vi "rs3 start all 2.vi"(7 "capacity":i32=2, 8 "error in (no error)":errorcluster, 9 "Count of Streams":i32=2, 10 "Sensor in":u64, 11 "Stream profile array":u64[](array[numeric])) -> (0 "error out":errorcluster, 2 "sensor out":u64, 3 "Config Error":string, 5 "queue out":u64)   [LabVIEW 2019, in "libRealSense3.lvlib"]
doc: "STARTs all the streams for the selected sensor.\n\nInput:\nStream profile array The array containing the handles to the Profiles you want to stream\nCount Number of streams in the array\nCapacity Should generally exceed or equal the count."
uses:
  libRealSense3.lvlib
panel:
  out "Sensor":dbl
  out "Stream Count":dbl
  # "RS3 Start all"
  # "(C) Intel Corp 2017,  AGJ"
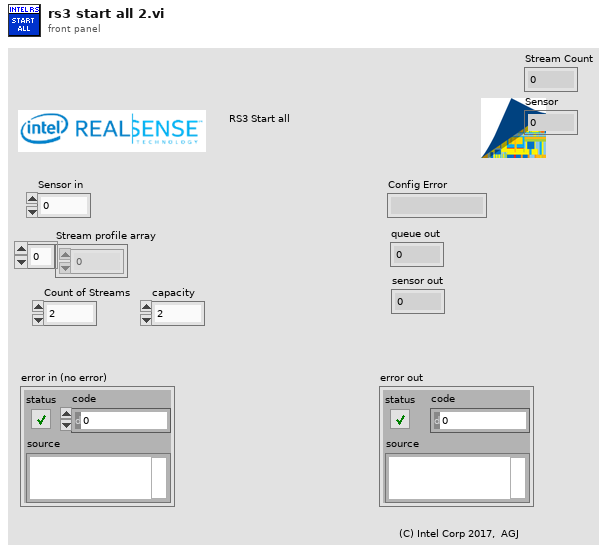
[diagram p1: front panel]
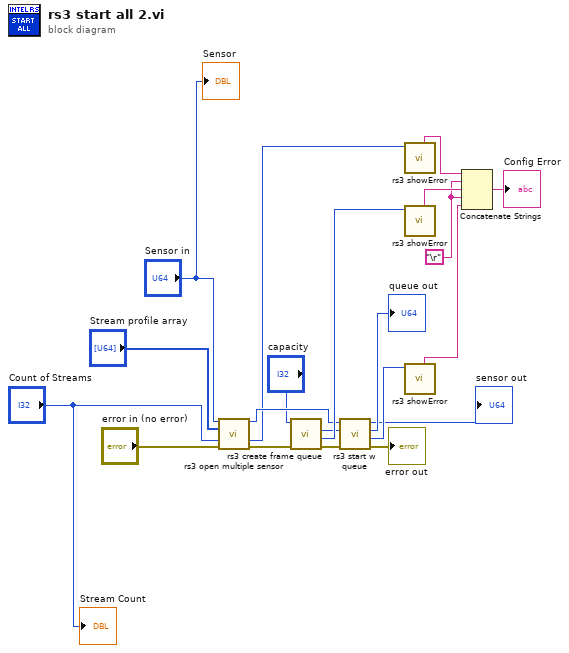
[diagram p0: block diagram]
diagram:
  w8 = "\r"
  n1 = call "rs3 open multiple sensor.vi"("sensor in"="Sensor in", "stream profile array"="Stream profile array", "Count of Streams"="Count of Streams", "error in (no error)"="error in (no error)") -> ("sensor out"=w15:u64, "error"=w13:u64, "error out"=w3:errorcluster)  [unwired: 9 in]
  n2 = call "rs3 create frame queue.vi"("error in (no error)"=w3, "capacity"="capacity") -> ("error out"=w14:errorcluster, "error"=w17:u64, "queue"=w16:u64)  [unwired: 7 in]
  n3 = call "rs3 start w queue.vi"("Sensor  in"=w15, "queue in"=w16, "error in (no error)"=w14) -> ("sensor out"=→"sensor out":u64, "queue out"=→"queue out":u64, "error"=w18:u64, "error out"=→"error out":errorcluster)  [unwired: 4 in]
  n4 = call "rs3 showError.vi"("error"=w13) -> ("Error summary"=w10:string)  [unwired: 6 in, 4 out]
  n5 = call "rs3 showError.vi"("error"=w17) -> ("Error summary"=w9:string)  [unwired: 6 in, 4 out]
  n6 = call "rs3 showError.vi"("error"=w18) -> ("Error summary"=w7:string)  [unwired: 6 in, 4 out]
  n7 = Concatenate Strings(w10, w8, w9, w8, w7) -> (→"Config Error":string)
  "Stream Count" <- "Count of Streams"
  "Sensor" <- "Sensor in"
